vi "Associate a File Extension.vi"(7 "Root Key(HKLM)":T1=enum."HKEY_LOCAL_MACHINE", 8 "error in (no error)":errorcluster, 10 ".ext":string=".myext", 11 "exe path":path) -> (0 "error out":errorcluster)   [LabVIEW 2014]
uses:
  <vilib>/registry/registry.llb/Registry RtKey.ctl
  <vilib>/registry/registry.llb/Write Registry Value Simple STR.vi
panel:
  in  "group":string="NEVSTOP"
  out "rootKey":string
  out "subkey":string
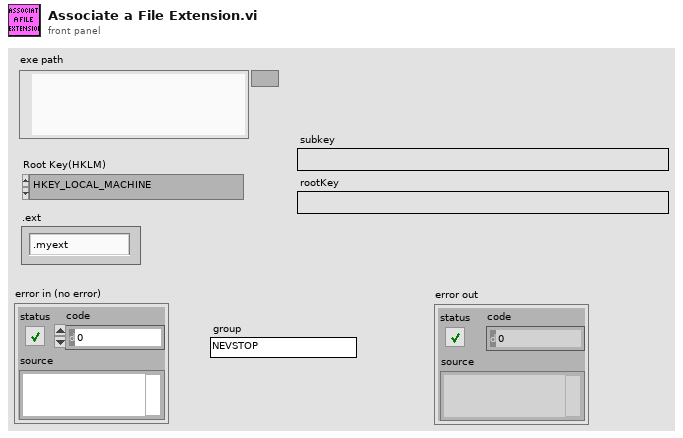
[diagram p1: front panel]
types:
  T1 = typedef "Registry RtKey.ctl" = enum32{"HKEY_CLASSES_ROOT", "HKEY_CURRENT_USER", "HKEY_LOCAL_MACHINE", "HKEY_USERS", "HKEY_PERFORMANCE_DATA", "HKEY_CURRENT_CONFIG", "HKEY_DYN_DATA"}
  T2 = typedef "Registry refnum.ctl" = refnum<k1>
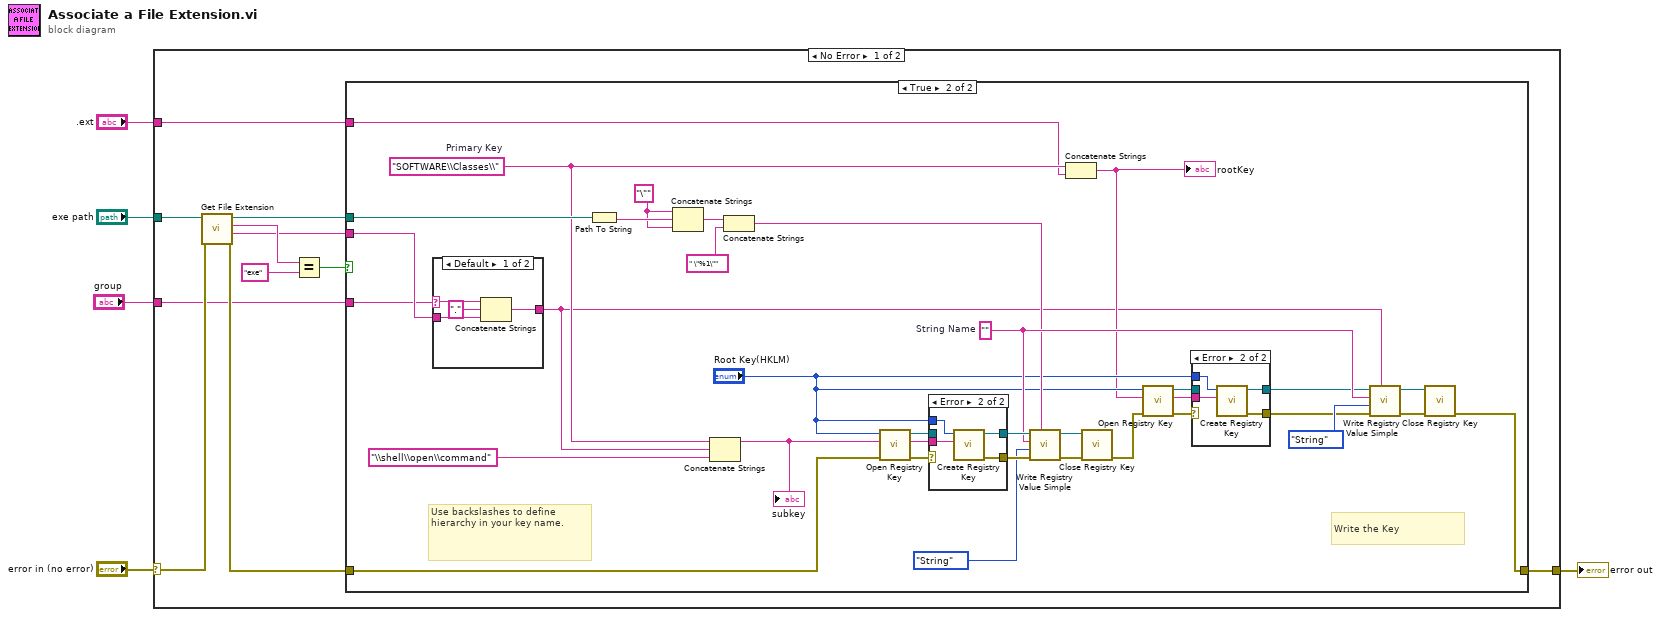
[diagram p0: block diagram]
diagram:
  n1 = case shown="No Error" "error in (no error)" {
    selector: "error in (no error)" -> [w12 w68]
    tunnel: [w16 w68] -> w5
    tunnel: "exe path" -> [w15 _]
    tunnel: "group" -> [w7 _]
    tunnel: ".ext" -> [w6 _]
    frame No Error {
      n2 = call <vilib>:"Get File Extension.vi"("error in (no error)"=w12, "file"=w15) -> ("error out"=w11:errorcluster, "filename without extension"=w8:string, "lowercase file extension"=w9:string, "dup file"=w10:path)  [unwired: 6 in]
      n3 = Equal?(x=w9, y="exe") -> (x = y?=w13:bool)
      n4 = case shown="True" w13 {
        tunnel: [w17 w41] -> w16
        tunnel: w11 -> [w17 w34]
        tunnel: w8 -> [_ w25]
        tunnel: w10 -> [_ w39]
        tunnel: w7 -> [_ w18]
        tunnel: w6 -> [_ w19]
        frame False {
        }
        frame True {
          w20 = "\"" ("string")
          w23 = "SOFTWARE\\Classes\\"  # Primary Key
          w40 = ""  # String Name
          # "Use backslashes to define hierarchy in your key name."
          # "Write the Key"
          n5 = case shown="Default" w18 {
            selector: w18 -> [w52 _]
            tunnel: w25 -> [w54 w55]
            tunnel: [w53 w55] -> w22
            frame Default {
              n6 = Concatenate Strings(w52, "." ("string"), w54) -> (w53:string)
            }
            frame "" {
            }
          }
          n7 = Path To String(path=w39) -> (string=w38:string)
          n8 = Concatenate Strings(w20, w38, w20) -> (w21:string)
          n9 = Concatenate Strings(w23, w22, "\\shell\\open\\command" ("subkey")) -> (w35:string)
          "subkey" <- w35
          n10 = Concatenate Strings(w21, " \"%1\"" ("string")) -> (w36:string)
          n11 = call <vilib>:"Open Registry Key.vi"("error in (no error)"=w34, "subkey"=w35, "root key (HKEY_LOCAL_MACHINE)"="Root Key(HKLM)") -> ("error out"=w33:errorcluster, "refnum out"=w32:T2)  [unwired: 7 in]
          n12 = case shown="Error" w33 {
            selector: w33 -> [w63 _]
            tunnel: [w63 w67] -> w49
            tunnel: [w62 w66] -> w47
            tunnel: "Root Key(HKLM)" -> [_ w65]
            tunnel: w35 -> [_ w64]
            tunnel: w32 -> [w62 _]
            frame No Error {
            }
            frame Error {
              n13 = call <vilib>:"Create Registry Key.vi"("subkey"=w64, "root key (HKEY_LOCAL_MACHINE)"=w65) -> ("error out"=w67:errorcluster, "refnum out"=w66:T2)  [unwired: 7 in, 1 out]
            }
          }
          n14 = call-poly <vilib>:"Write Registry Value Simple.vi"("String/Binary data"=w36, "error in (no error)"=w49, "simple data type"=enum16{"String", "Binary", "DWORD"}."String", "value"=w40, "refnum"=w47) -> ("error out"=w45:errorcluster, "refnum out"=w46:T2)  [unwired: 3 in]
          n15 = Concatenate Strings(w23, w19) -> (w24:string)
          "rootKey" <- w24
          n16 = call <vilib>:"Close Registry Key.vi"("error in (no error)"=w45, "refnum"=w46) -> ("error out"=w26:errorcluster)  [unwired: 5 in]
          n17 = call <vilib>:"Open Registry Key.vi"("error in (no error)"=w26, "subkey"=w24, "root key (HKEY_LOCAL_MACHINE)"="Root Key(HKLM)") -> ("error out"=w30:errorcluster, "refnum out"=w31:T2)  [unwired: 7 in]
          n18 = case shown="Error" w30 {
            selector: w30 -> [w57 _]
            tunnel: [w57 w61] -> w29
            tunnel: [w56 w60] -> w28
            tunnel: "Root Key(HKLM)" -> [_ w59]
            tunnel: w24 -> [_ w58]
            tunnel: w31 -> [w56 _]
            frame No Error {
            }
            frame Error {
              n19 = call <vilib>:"Create Registry Key.vi"("subkey"=w58, "root key (HKEY_LOCAL_MACHINE)"=w59) -> ("error out"=w61:errorcluster, "refnum out"=w60:T2)  [unwired: 7 in, 1 out]
            }
          }
          n20 = call-poly <vilib>:"Write Registry Value Simple.vi"("String/Binary data"=w22, "error in (no error)"=w29, "simple data type"=enum16{"String", "Binary", "DWORD"}."String", "value"=w40, "refnum"=w28) -> ("error out"=w44:errorcluster, "refnum out"=w43:T2)  [unwired: 3 in]
          n21 = call <vilib>:"Close Registry Key.vi"("error in (no error)"=w44, "refnum"=w43) -> ("error out"=w41:errorcluster)  [unwired: 5 in]
        }
      }
    }
    frame Error {
    }
  }
  "error out" <- w5
